vi "SpeedCtrl_4B.vi"(5 "Reset":bool, 6 "dt (s)":dbl=-1.0 format="%.3f", 7 "PID gains":T2={"proportional gain (Kc)"=1.0, "integral time (Ti, min)"=0.0, "derivative time (Td, min)"=0.005} {"derivative time (Td, min)" format="%.5f"; "integral time (Ti, min)" format="%.3f"; "proportional gain (Kc)" format="%.3f"}, 8 "error in":errorcluster, 9 "Target Spd. \nmm/s":T3, 10 "Speed Now":T1, 11 "Enable":bool) -> (0 "error out":errorcluster)   [LabVIEW 2018]
doc: "The myRIO Project template acquires acceleration data from the onboard accelerometer and displays the changes of acceleration values in a waveform chart."
uses:
  <vilib>/myRIO/Express VI/Onboard IO/PWM/PWM Express VI.xnode
  <vilib>/myRIO/Common/Instrument Driver Framework/Utilities/typedefs/Generic FPGA Reference.ctl
  <vilib>/myRIO/Common/Instrument Driver Framework/Utilities/typedefs/myRIO v1.0 Reference.ctl
  <vilib>/myRIO/Common/Instrument Driver Framework/Utilities/typedefs/Hardware Version Enum.ctl
  <vilib>/myRIO/Common/Instrument Driver Framework/Utilities/typedefs/myRIO Generic Hardware Reference.ctl
  <vilib>/myRIO/Common/Instrument Driver Framework/Utilities/vis/Is FPGA Ref Available.vi
  <vilib>/userdefined/High Color/nirio_resource_hc.ctl
  <vilib>/myRIO/Express VI/Onboard IO/DO/DO Express VI.xnode
  <vilib>/myRIO/Instrument Drivers/Onboard IO/DIO/vis/Write.vi
  <vilib>/myRIO/Instrument Drivers/Onboard IO/DIO/DIO.lvlib
  <vilib>/myRIO/Common/Instrument Driver Framework/myRIO v1.0/DIO/typedefs/DIO Channels Enum.ctl
  <vilib>/myRIO/Common/Instrument Driver Framework/myRIO v1.0/DIO/typedefs/DIO Channels List.ctl
  <vilib>/myRIO/Instrument Drivers/Onboard IO/DIO/typedefs/DIO Reference.ctl
  <vilib>/myRIO/Instrument Drivers/Onboard IO/DIO/vis/myRIO DIO Open.xnode
  <vilib>/myRIO/Common/Instrument Driver Framework/myRIO v1.0/DIO/vis/myRIO v1.1 Open DIO.vi
  <vilib>/myRIO/Instrument Drivers/Onboard IO/PWM/vis/Set Duty Cycle and Frequency.vi
  <vilib>/myRIO/Instrument Drivers/Onboard IO/PWM/PWM.lvlib
  <vilib>/myRIO/Instrument Drivers/Onboard IO/PWM/typedefs/PWM Configuration.ctl
  <vilib>/myRIO/Common/Instrument Driver Framework/myRIO v1.0/PWM/typedefs/PWM Channels Enum.ctl
  <vilib>/myRIO/Instrument Drivers/Onboard IO/PWM/typedefs/PWM Reference.ctl
  <vilib>/myRIO/Instrument Drivers/Onboard IO/PWM/vis/myRIO PWM Open.xnode
  <vilib>/myRIO/Common/Instrument Driver Framework/myRIO v1.0/PWM/vis/myRIO v1.1 Open PWM.vi
  <vilib>/addons/control/pid/NI_PID_pid.lvlib
  <vilib>/addons/control/pid/pid.llb/PID (DBL).vi
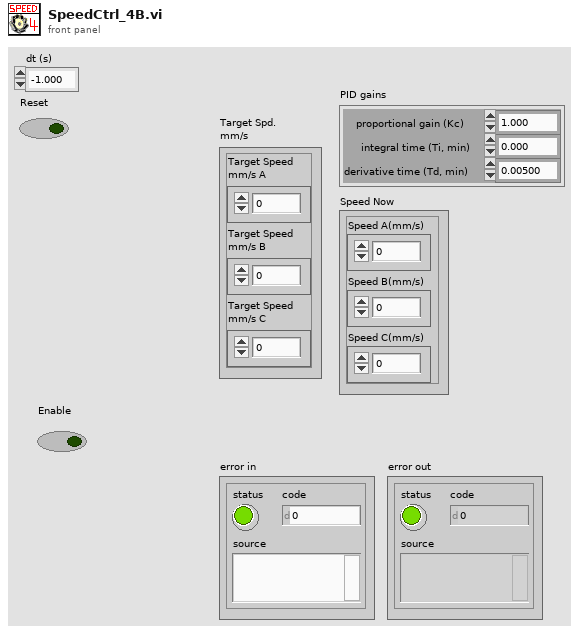
[diagram p1: front panel]
types:
  T1 = cluster{"Speed A(mm/s)":dbl, "Speed B(mm/s)":dbl, "Speed C(mm/s)":dbl}
  T2 = cluster{"proportional gain (Kc)":dbl, "integral time (Ti, min)":dbl, "derivative time (Td, min)":dbl}
  T3 = cluster{"Target Speed\nmm/s A":dbl, "Target Speed\nmm/s B":dbl, "Target Speed\nmm/s C":dbl}
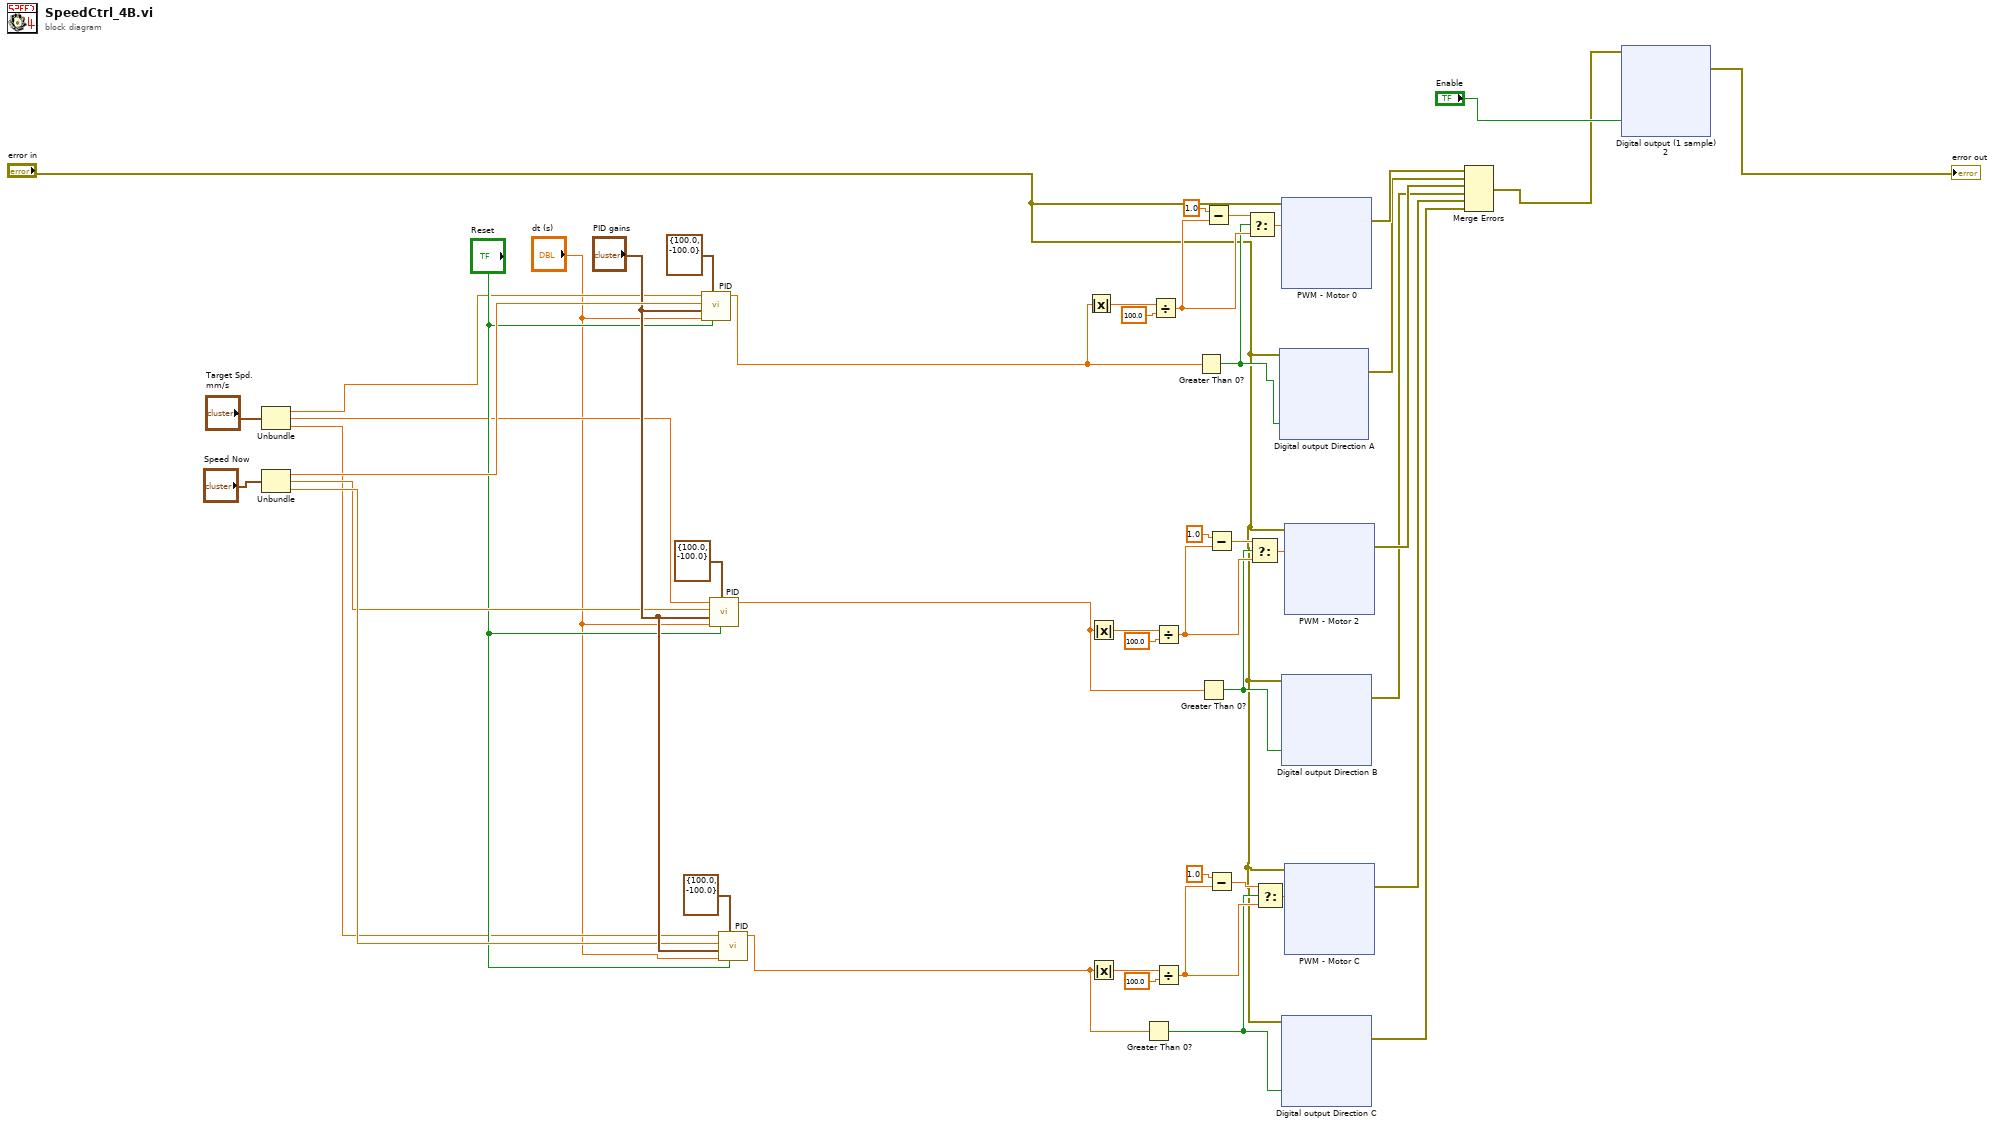
[diagram p0: block diagram]
diagram:
  n1 = Unbundle("Target Spd. \nmm/s") -> ("Target Speed\nmm/s A"=w7:dbl, "Target Speed\nmm/s B"=w6:dbl, "Target Speed\nmm/s C"=w5:dbl)
  n2 = Unbundle("Speed Now") -> ("Speed A(mm/s)"=w14:dbl, "Speed B(mm/s)"=w9:dbl, "Speed C(mm/s)"=w10:dbl)
  n3 = call-poly <vilib>:"PID.vi"("reinitialize? (F)"="Reset", "output range"=cluster{"output high":dbl, "output low":dbl} {"output high"=100.0, "output low"=-100.0}, "dt (s)"="dt (s)", "PID gains"="PID gains", "process variable"=w14, "setpoint"=w7) -> ("output"=w3:dbl)  [unwired: 4 in, 1 out]
  n4 = call-poly <vilib>:"PID.vi"("reinitialize? (F)"="Reset", "output range"=cluster{"output high":dbl, "output low":dbl} {"output high"=100.0, "output low"=-100.0}, "dt (s)"="dt (s)", "PID gains"="PID gains", "process variable"=w9, "setpoint"=w6) -> ("output"=w4:dbl)  [unwired: 4 in, 1 out]
  n5 = call-poly <vilib>:"PID.vi"("reinitialize? (F)"="Reset", "output range"=cluster{"output high":dbl, "output low":dbl} {"output high"=100.0, "output low"=-100.0}, "dt (s)"="dt (s)", "PID gains"="PID gains", "process variable"=w10, "setpoint"=w5) -> ("output"=w2:dbl)  [unwired: 4 in, 1 out]
  n6 = Absolute Value(x=w3) -> (abs(x)=w44:dbl)
  n7 = Absolute Value(x=w4) -> (abs(x)=w36:dbl)
  n8 = Absolute Value(x=w2) -> (abs(x)=w30:dbl)
  n9 = Greater Than 0?(x=w2) -> (x > 0?=w24:bool)
  n10 = Divide(x=w44, y=100.0) -> (x/y=w41:dbl)
  n11 = Divide(x=w36, y=100.0) -> (x/y=w38:dbl)
  n12 = Divide(x=w30, y=100.0) -> (x/y=w28:dbl)
  n13 = Greater Than 0?(x=w3) -> (x > 0?=w26:bool)
  n14 = Greater Than 0?(x=w4) -> (x > 0?=w25:bool)
  n15 = Subtract(x=1.0, y=w41) -> (x-y=w40:dbl)
  n16 = Subtract(x=1.0, y=w38) -> (x-y=w39:dbl)
  n17 = Subtract(x=1.0, y=w28) -> (x-y=w27:dbl)
  n18 = Select(t=w40, s=w26, f=w41) -> (s? t:f=w45:dbl)
  n19 = Select(t=w39, s=w25, f=w38) -> (s? t:f=w35:dbl)
  n20 = Select(t=w27, s=w24, f=w28) -> (s? t:f=w31:dbl)
  n21 = xnode "Digital output Direction A"("DIRA (A/DIO13 (Pin 26))"=w26, "error in (no error)"="error in") -> ("error out"=w47:errorcluster)
  n22 = xnode "PWM - Motor 0"("Duty Cycle"=w45, "error in (no error)"="error in") -> ("error out"=w48:errorcluster)
  n23 = xnode "Digital output Direction B"("DIRB (B/DIO13 (Pin 26))"=w25, "error in (no error)"="error in") -> ("error out"=w22:errorcluster)
  n24 = xnode "Digital output Direction C"("DIRC (C/DIO1 (DIO1))"=w24, "error in (no error)"="error in") -> ("error out"=w20:errorcluster)
  n25 = xnode "PWM - Motor 2"("Duty Cycle"=w35, "error in (no error)"="error in") -> ("error out"=w23:errorcluster)
  n26 = xnode "PWM - Motor C"("Duty Cycle"=w31, "error in (no error)"="error in") -> ("error out"=w21:errorcluster)
  n27 = Merge Errors(w48, w47, w23, w22, w21, w20) -> (w33:errorcluster)
  n28 = xnode "Digital output (1 sample) 2"("ENABLE (A/DIO4 (Pin 19))"="Enable", "error in (no error)"=w33) -> ("error out"=→"error out":errorcluster)
